vi "ResetQuadrature.vi"() -> ()   [LabVIEW 2016]
panel:
  in  "Current Pulse Width":dbl format="%#_13g"
  in  "Current Quadrature":dbl format="%#_13g"
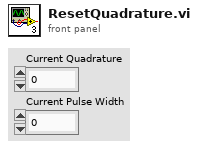
[diagram p1: front panel]
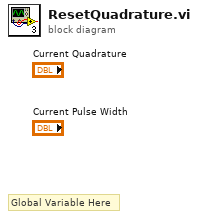
[diagram p0: block diagram]
diagram:
  # "Global Variable Here"
